vi "Write Settings.vi"(8 "error in (no error)":errorcluster, 10 "Settings":T1={"Integration Time (ms)"=80, "Temp  Compensation "=FALSE, "Optical Smoothing Level"=0, "Number of Scans to Average"=1, "Digitizer Clock Rate Setting"=3} {"Digitizer Clock Rate Setting" min=1 max=3; "Number of Scans to Average" min=1 max=10000 step=1; "Optical Smoothing Level" min=0 max=4 step=1}, 11 "StellarNetSpectrometer in":refnum<class "StellarNetSpectrometer.lvclass">) -> (0 "error out":errorcluster, 3 "StellarNetSpectrometer out":refnum<class "StellarNetSpectrometer.lvclass">)   [LabVIEW 2013, in "StellarNetSpectrometer.lvclass"]
uses:
  StellarNetSpectrometer.lvclass
  StellarNetSpectrometer.lvclass/StellarNetSpectrometer.ctl
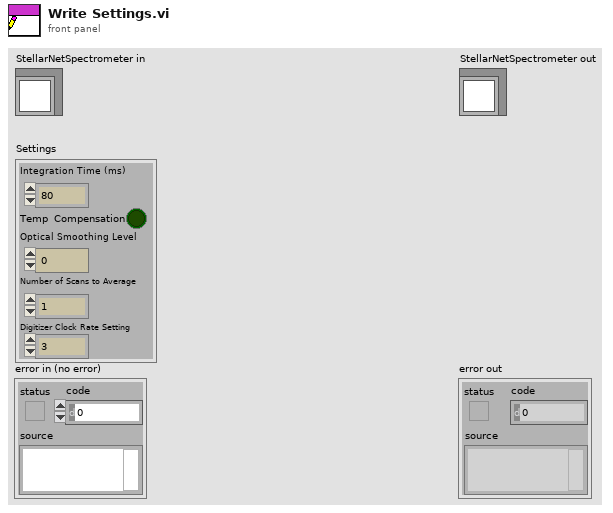
[diagram p1: front panel]
types:
  T1 = cluster{"Integration Time (ms)":i32, "Temp  Compensation ":bool, "Optical Smoothing Level":i32, "Number of Scans to Average":i32, "Digitizer Clock Rate Setting":i32}
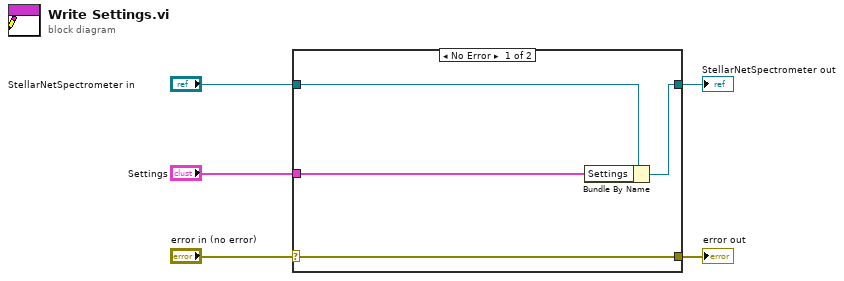
[diagram p0: block diagram]
diagram:
  n1 = case shown="No Error" "error in (no error)" {
    selector: "error in (no error)" -> [w9 w10]
    tunnel: [w9 w10] -> w4
    tunnel: [w7 w11] -> w2
    tunnel: "StellarNetSpectrometer in" -> [w8 w11]
    tunnel: "Settings" -> [w6 _]
    frame No Error {
      n2 = Bundle By Name(cluster=w8, "Settings"=w6) -> (w7:refnum<class "StellarNetSpectrometer.lvclass">)
    }
    frame Error {
    }
  }
  "error out" <- w4
  "StellarNetSpectrometer out" <- w2
